vi "MOTOR MCP SPI.vi"(3 "Data to Write":u8[](array[numeric])=[0, 0, 0, 0, 0, 0, 0, 0, 0, 0] format="%x", 4 "Frames to Write":u8, 5 "SPI Config In":T1) -> (0 "Data Read":u8[](array[numeric]) format="%x", 1 "Frames Read":u8, 2 "SPI Config Out":T1)   [LabVIEW 2019]
uses:
  SPI Config.ctl
  <vilib>/Platform/TimedLoop/XDataNode/timing_clust.ctl
  <vilib>/Platform/TimedLoop/XDataNode/nitl_modes.ctl
  <vilib>/Platform/TimedLoop/XDataNode/wakeup.ctl
  <vilib>/rvi/Emulation/niFpgaSctlEmulationGetInTimedLoop.vi
  <vilib>/rvi/Emulation/niFpgaEmulationReportErrorSimple.vi
  <vilib>/rvi/Emulation/niFpgaGetClockAttributes.vi
  <vilib>/rvi/Emulation/niFpgaCriticalErrorInLSC.vi
  <vilib>/rvi/eio/common/nirviEmuTemplateMethod_errors.vi
  <vilib>/platform/TimedLoop/XDataNode/XDataNode.xnode
  <vilib>/eio/EIONode/EIONode.xnode
  <vilib>/Platform/TimedLoop/XDataNode/XDNodeRunTimeDep.lvlib
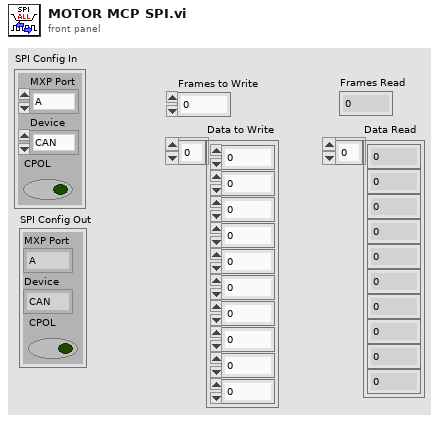
[diagram p1: front panel]
types:
  T1 = typedef "SPI Config.ctl" = cluster{"MXP Port":enum16{"A", "B"}, "Device":enum16{"CAN", "ENC", "IMU1", "IMU2"}, "CPOL":bool}
  T2 = typedef "XDNodeRunTimeDep.lvlib/timing_clust.ctl" = cluster{"Expected End [f-1]":u64, "Actual End [f-1]":u64, "Finished Late? [f-1]":bool, "Expected End [i-1]":u64, "Actual End [i-1]":u64, "Finished Late? [i-1]":bool, "Expected Start [i]":u64, "Actual Start [i]":u64, "Expected Start [f]":u64, "Actual Start [f]":u64, "Source Name":string, "Structure Name":string, "Period":i64, "Deadline":i64, "Offset":i64, "Start":i64, "Priority":i32, "Timeout":i32, "Mode":T3, "Wakeup Reason":T4, "Error":errorcluster, "Source Type":string, "Secondary Source Type":string, "Global End Time":u64, "Global Start Time":u64, "Frame Duration":u64, "Iteration Duration":u64, "Assigned CPU":i32, "I/O Scan Engine Mode":u32}
  T3 = typedef "XDNodeRunTimeDep.lvlib/nitl_modes.ctl" = enum32{"No Change", "Process missed periods, maintain original phase", "Discard missed periods, maintain original phase", "Process missed periods, ignore original phase", "Discard missed periods, ignore original phase"}
  T4 = typedef "XDNodeRunTimeDep.lvlib/wakeup.ctl" = enum32{"Normal", "Aborted", "Asynchronous wakeup", "Timing source error", "Timed loop error", "Timeout"}
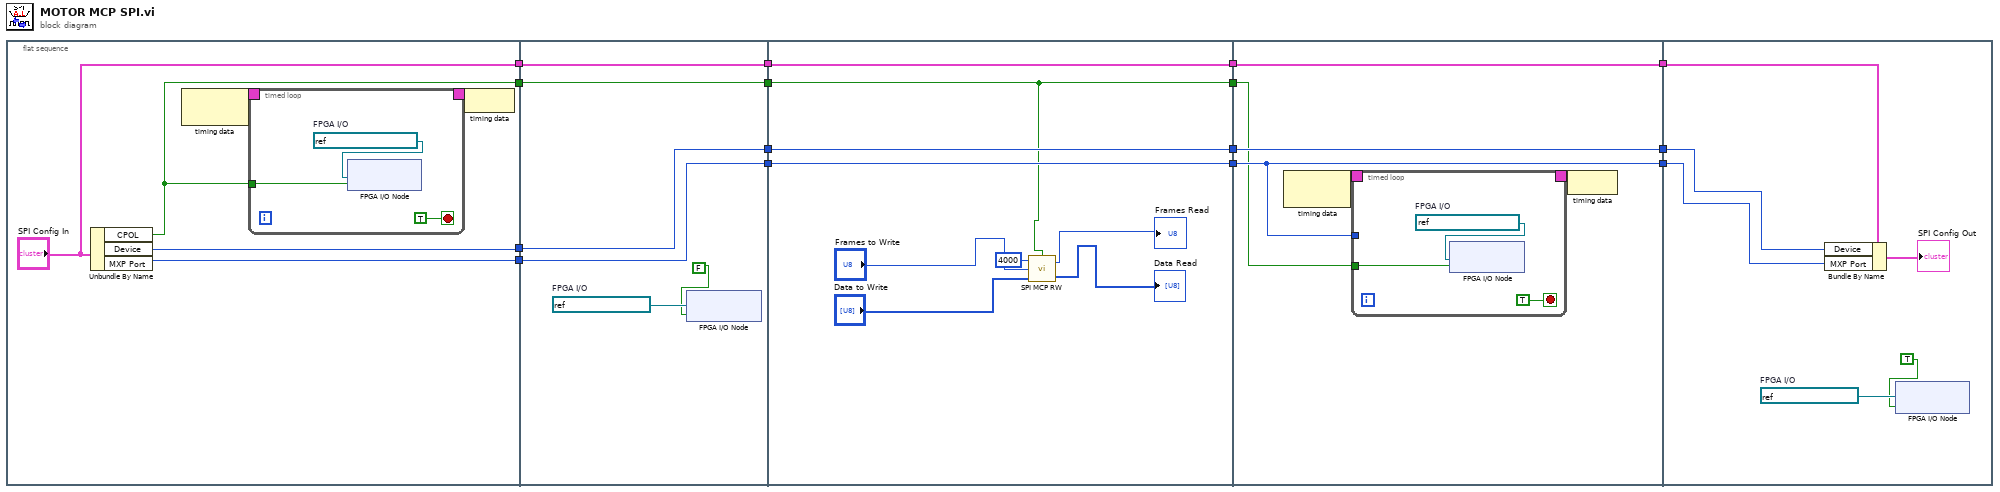
[diagram p0: block diagram]
diagram:
  n1 = flat-sequence {
    tunnel: ["SPI Config In"] -> w12
    tunnel: [w20] -> w11
    tunnel: [w17] -> w10
    tunnel: [w16] -> w8
    tunnel: [w29] -> w15
    tunnel: [w30] -> w14
    tunnel: [w34] -> w13
    tunnel: w12 -> [w34]
    tunnel: w11 -> [w30]
    tunnel: w10 -> [w29]
    tunnel: [w33] -> w9
    tunnel: w8 -> [w33]
    tunnel: w15 -> [w43]
    tunnel: [w43] -> w7
    tunnel: [w42] -> w5
    tunnel: w14 -> [w42]
    tunnel: w13 -> [w41]
    tunnel: [w41] -> w3
    tunnel: w9 -> [w40]
    tunnel: [w40] -> w1
    tunnel: w7 -> [w45]
    tunnel: [w45] -> w6
    tunnel: w5 -> [w49]
    tunnel: [w49] -> w4
    tunnel: w3 -> [w48]
    tunnel: [w48] -> w2
    tunnel: w1 -> [w44]
    tunnel: w6 -> [w60]
    tunnel: w4 -> [w61]
    tunnel: w2 -> [w62]
    frame #0 {
      n2 = Unbundle By Name("SPI Config In") -> ("CPOL"=w16:bool, "Device"=w20:enum16{"CAN", "ENC", "IMU1", "IMU2"}, "MXP Port"=w17:enum16{"A", "B"})
      n3 = node-c288() -> (w19:T2)  [unwired: 1 in]
      n4 = timed-loop {
        timing: w19 -> [_]
        timing-out: [_] -> w18
        tunnel: w16 -> [w23]
        stop <- TRUE stop-if-true
        w22 = refnum<k21> "MOTOR MCP CLK"  # FPGA I/O
        n5 = xnode "FPGA I/O Node"("I/O Item"=w23, "FPGA I/O In"=w22) -> ()  [unwired: 1 out]
      }
      n6 = node-c288(w18) -> ()
    }
    frame #1 {
      w32 = refnum<k21> "MOTOR MCP CS"  # FPGA I/O
      n7 = xnode "FPGA I/O Node"("I/O Item"=FALSE ("Value"), "FPGA I/O In"=w32) -> ()  [unwired: 1 out]
    }
    frame #2 {
      n8 = call "SPI MCP RW.vi"("CPOL"=w40, "Data to Write"="Data to Write", "Frames to Write"="Frames to Write", "SPI Frequency (KHz)"=u16 4000) -> ("Data Read"=→"Data Read":u8[], "Frames Read"=→"Frames Read":u8)
    }
    frame #3 {
      n9 = node-c288() -> (w47:T2)  [unwired: 1 in]
      n10 = timed-loop {
        timing: w47 -> [_]
        timing-out: [_] -> w46
        tunnel: w45 -> [_]
        tunnel: w44 -> [w51]
        stop <- TRUE stop-if-true
        w50 = refnum<k21> "MOTOR MCP CLK"  # FPGA I/O
        n11 = xnode "FPGA I/O Node"("I/O Item"=w51, "FPGA I/O In"=w50) -> ()  [unwired: 1 out]
      }
      n12 = node-c288(w46) -> ()
    }
    frame #4 {
      w58 = refnum<k21> "MOTOR MCP CS"  # FPGA I/O
      n13 = Bundle By Name(cluster=w62, "Device"=w61, "MXP Port"=w60) -> (→"SPI Config Out":T1)
      n14 = xnode "FPGA I/O Node"("I/O Item"=TRUE ("Value"), "FPGA I/O In"=w58) -> ()  [unwired: 1 out]
    }
  }
